vi "TestComplete.vi"(8 "error in (no error)":errorcluster, 10 "Done":bool, 11 "TestBench in":refnum<class "TestBench.lvclass">) -> (0 "error out":errorcluster, 3 "TestBench out":refnum<class "TestBench.lvclass">)   [LabVIEW 2019, in "TestBench.lvlib" / "TestBench.lvclass"]
uses:
  TestBench.lvclass
  C:/Program Files (x86)/National Instruments/LabVIEW 2019/vi.lib/ActorFramework/Actor/Actor.lvclass
  <vilib>/ActorFramework/Actor/Actor.lvclass/Actor.ctl
  <vilib>/ActorFramework/Message Enqueuer/Message Enqueuer.lvclass/Message Enqueuer.ctl
  TestBench.lvclass/TestBench.ctl
  <vilib>/NI/Event Source Actor/Event Source/Event Source Messages/Unregister Msg/Unregister Msg.lvclass/Unregister Msg.ctl
  UnitTestEngine/UnitTestEngine Messages/TestComplete Msg/TestComplete Msg.lvclass/TestComplete Msg.ctl
  fcf2d937-4a27-4573-94ea-ac01c026fc21.vi
  <vilib>/ActorFramework/Message Enqueuer/Init from Existing Queue.vi
  <vilib>/ActorFramework/Message Enqueuer/Enqueue.vi
  <vilib>/NI/Event Source Actor/Event Source/Event Source Messages/Unregister Msg/Unregister Msg.lvclass
  C:/Program Files (x86)/National Instruments/LabVIEW 2019/vi.lib/ActorFramework/Message/Message.lvclass
  <vilib>/ActorFramework/Stop Msg/Stop Msg.lvclass
  UnitTestEngine/UnitTestEngine Messages/TestComplete Msg/TestComplete Msg.lvclass
  <vilib>/ActorFramework/Message Priority Queue/Priority Enqueue.vi
  <vilib>/ActorFramework/Message Enqueuer/Message Enqueuer.lvclass
  <vilib>/ActorFramework/Actor/Actor.lvclass
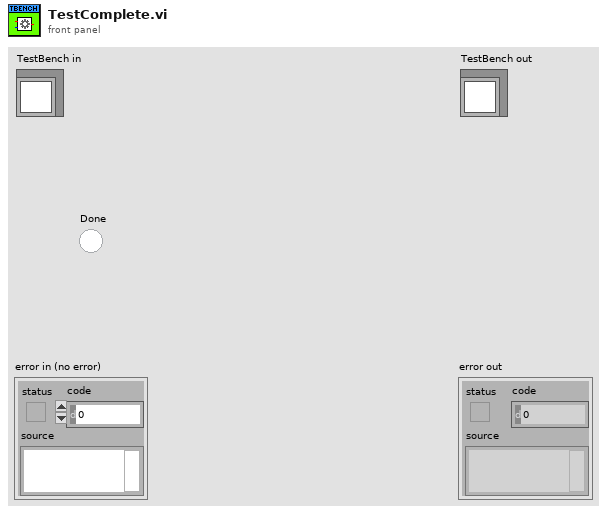
[diagram p1: front panel]
types:
  T1 = map{string, refnum<class "Message Enqueuer.lvclass">}
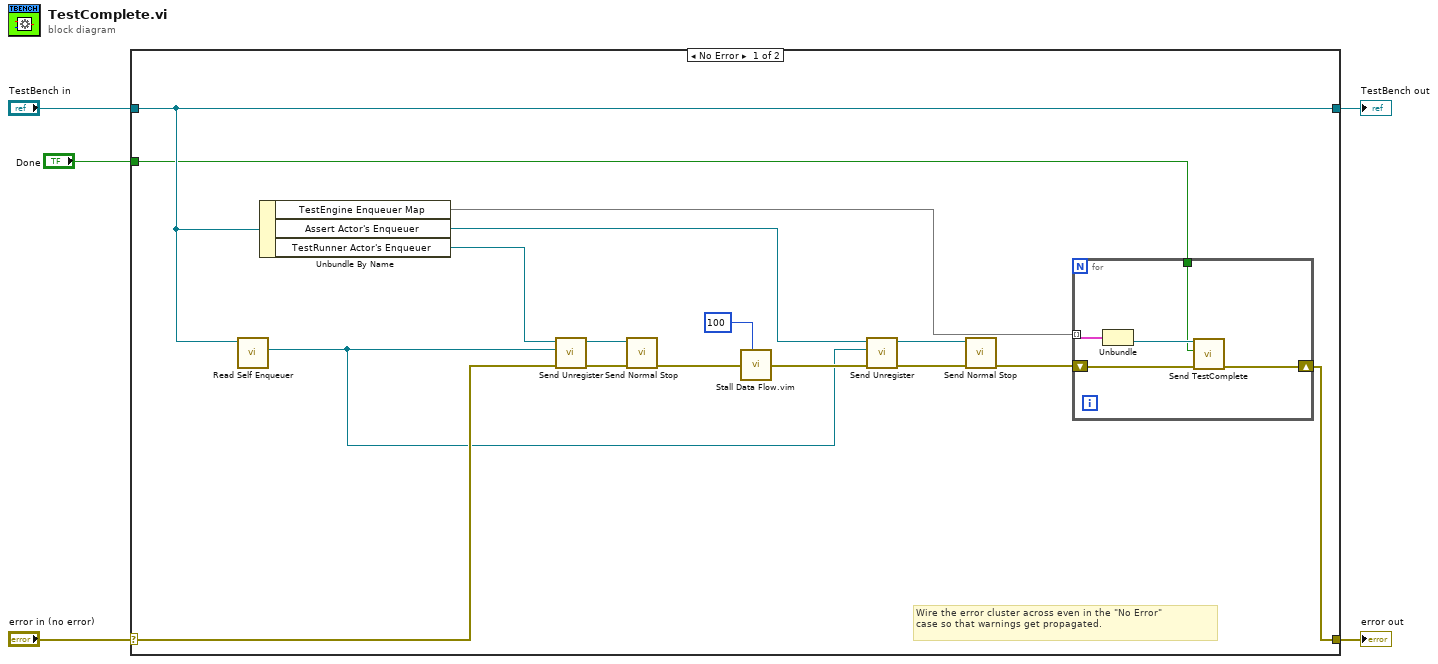
[diagram p0: block diagram]
diagram:
  n1 = case shown="No Error" "error in (no error)" {
    selector: "error in (no error)" -> [w15 w28]
    tunnel: [w11 w28] -> w4
    tunnel: [w16 w27] -> w2
    tunnel: "TestBench in" -> [w16 w27]
    tunnel: "Done" -> [w13 _]
    frame No Error {
      # "Wire the error cluster across even in the \"No Error\"\ncase so that warnings get propagated."
      n2 = call <vilib>:"Read Self Enqueuer.vi"("Actor"=w16) -> ("Self Enqueuer"=w6:refnum<class "Message Enqueuer.lvclass">)  [unwired: 10 in]
      n3 = Unbundle By Name(w16) -> ("TestEngine Enqueuer Map"=w14:T1, "Assert Actor's Enqueuer"=w10:refnum<class "Message Enqueuer.lvclass">, "TestRunner Actor's Enqueuer"=w21:refnum<class "Message Enqueuer.lvclass">)
      n4 = call <vilib>:"Send Unregister.vi"("Error In"=w15, "Registrant Address"=w6, "Event Source Address"=w21) -> ("Error Out"=w19:errorcluster, "Event Source Address Out"=w20:refnum<class "Message Enqueuer.lvclass">)  [unwired: 7 in]
      n5 = call <vilib>:"Send Normal Stop.vi"("error in (no error)"=w19, "Message Enqueuer"=w20) -> ("error out"=w18:errorcluster)  [unwired: 9 in]
      n6 = call "Stall Data Flow.vim"("value in"=w18, "milliseconds to wait"=u32 100) -> ("value out"=w7:errorcluster)  [unwired: 1 out]
      n7 = call <vilib>:"Send Unregister.vi"("Error In"=w7, "Registrant Address"=w6, "Event Source Address"=w10) -> ("Error Out"=w8:errorcluster, "Event Source Address Out"=w9:refnum<class "Message Enqueuer.lvclass">)  [unwired: 7 in]
      n8 = call <vilib>:"Send Normal Stop.vi"("error in (no error)"=w8, "Message Enqueuer"=w9) -> ("error out"=w12:errorcluster)  [unwired: 9 in]
      n9 = for {
        tunnel: w14 -> [w26] mode=indexing
        tunnel: w13 -> [w24]
        shift-right: [w22] -> w11
        shift-left: w12 -> [w23]
        n10 = Unbundle(w26) -> ("TestEngine Actor's Enqueuer"=w25:refnum<class "Message Enqueuer.lvclass">)  [unwired: 1 out]
        n11 = call "Send TestComplete.vi"("error in (no error)"=w23, "Done"=w24, "Message Enqueuer"=w25) -> ("error out"=w22:errorcluster)  [unwired: 7 in, 1 out]
      }
    }
    frame Error {
    }
  }
  "error out" <- w4
  "TestBench out" <- w2
